vi "Searching Algorithm.vi"(7 "Input String":string, 8 "Find":string, 10 "Start Index":u32) -> (0 "Done?":bool, 1 "Start of Find":u32, 2 "End of Find":u32, 5 "After Match":string)   [LabVIEW 2014]
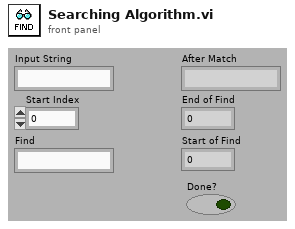
[diagram p1: front panel]
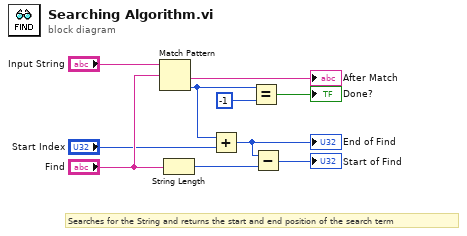
[diagram p0: block diagram]
diagram:
  # "Searches for the String and returns the start and end position of the search term"
  n1 = Match Pattern(string="Input String", regular expression="Find") -> (after substring=→"After Match":string, offset past match=w6:i32)  [unwired: 1 in, 2 out]
  n2 = String Length(string="Find") -> (length=w5:i32)
  n3 = Add(x=w6, y="Start Index") -> (x+y=w9:u32)
  "End of Find" <- w9
  n4 = Equal?(x=w6, y=-1) -> (x = y?=→"Done?":bool)
  n5 = Subtract(x=w9, y=w5) -> (x-y=→"Start of Find":u32)
